vi "PicoScope2000aSetupStreaming.vi"(0 "error in":errorcluster, 1 "Device Info":T1, 2 "handle in":i16, 3 "Acquisition Settings":T3={"Auto Stop"=FALSE, "Desired Sample Interval"=4, "Pre-trigger Samples"=0, "Post-trigger Samples"=1000, "Down-Sample Ratio"=1, "Down-Sample Mode"=0, "Time Units"=2} {"Time Units" items=["Nanoseconds (ns)"=2, "Microseconds (us)"=3, "Milliseconds (ms)"=4, "Seconds (s)"=5]; "Down-Sample Mode" items=["None"=0, "Aggregate"=1, "Decimate"=2, "Average"=4]}, 4 "Buffer and Transfer Settings":T2={"startIndex"=0, "Samples"=1000000, "Down Sample Ratio"=1, "Down-Sample Mode"=0} {"Down-Sample Mode" items=["None"=0, "Aggregate"=1, "Decimate"=2, "Average"=4]; "Down Sample Ratio" step=1; "Samples" format="%_6p"}, 5 "enabled array":i16[](array[numeric]), 10 "Pointers In":u64[][](array[numeric])) -> (11 "Pointer array":u64[][](array[numeric]), 14 "error out":errorcluster, 16 "handle out":i16, 17 "Sample Interval":u32, 19 "sampleIntervalTimeUnits":u32)   [LabVIEW 2010]
doc: "Set up the data buffers and calls RunStreaming to start the device streaming.\nData will be copied from the driver buffers into the corresponding application buffers using the wrapper dll."
uses:
  ps2000aWrap.dll
  ps2000a.dll
panel:
  # "Overview Buffer Size is the size of the temporary buffers used to\nstore data before returning it to the application."
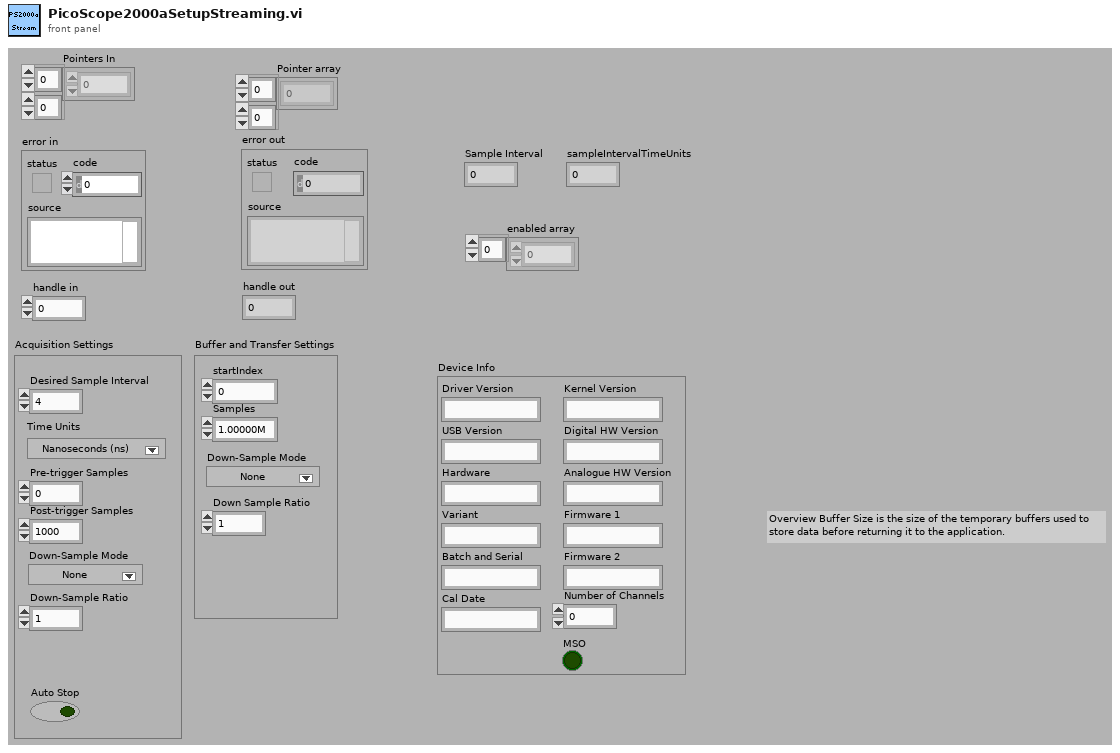
[diagram p1: front panel]
types:
  T1 = cluster{"Driver Version":string, "USB Version":string, "Hardware":string, "Variant":string, "Batch and Serial":string, "Cal Date":string, "Kernel Version":string, "Digital HW Version":string, "Analogue HW Version":string, "Firmware 1":string, "Firmware 2":string, "MSO":bool, "Number of Channels":i16}
  T2 = cluster{"startIndex":u64, "Samples":u64, "Down Sample Ratio":u64, "Down-Sample Mode":u32}
  T3 = cluster{"Auto Stop":bool, "Desired Sample Interval":u32, "Pre-trigger Samples":u32, "Post-trigger Samples":u32, "Down-Sample Ratio":u32, "Down-Sample Mode":i32, "Time Units":u32}
  T4 = cluster{"status":bool, "code":u32, "source":string}
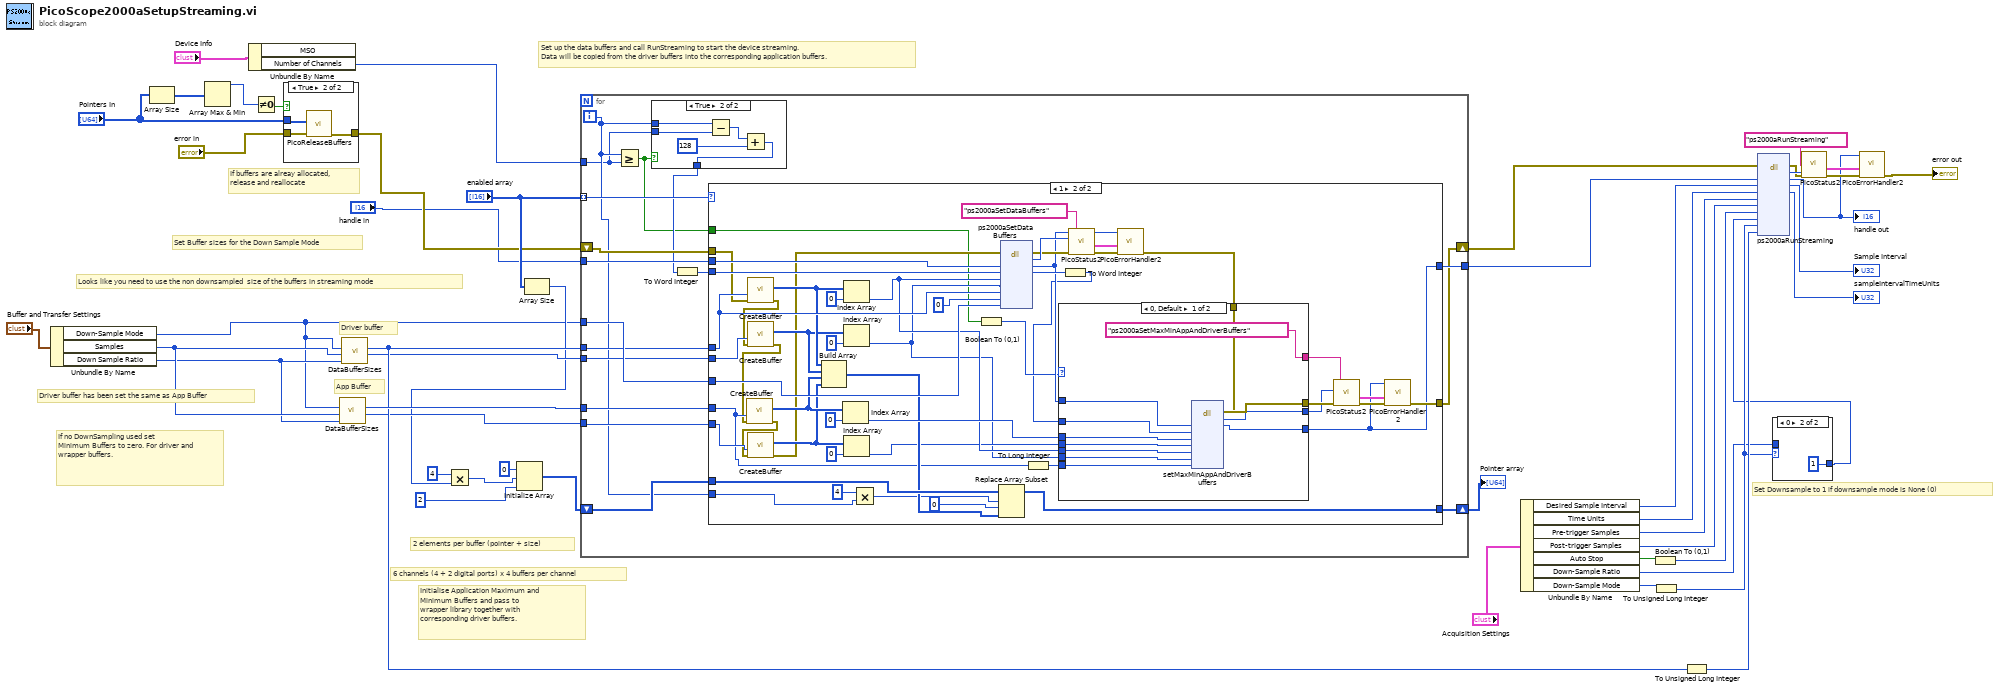
[diagram p0: block diagram]
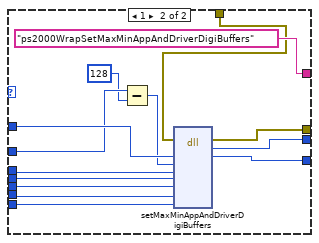
[diagram p6: hidden frame]
diagram:
  # "Set Downsample to 1 if downsample mode is None (0)"
  # "Looks like you need to use the non downsampled  size of the buffers in streaming mode"
  # "If buffers are alreay allocated,\nrelease and reallocate"
  # "2 elements per buffer (pointer + size)"
  # "6 channels (4 + 2 digital ports) x 4 buffers per channel"
  # "App Buffer"
  # "Driver buffer"
  # "Driver buffer has been set the same as App Buffer"
  # "Set Buffer sizes for the Down Sample Mode"
  # "If no DownSampling used set \nMinimum Buffers to zero. For driver and wrapper buffers."
  # "Initialise Application Maximum and\nMinimum Buffers and pass to \nwrapper library together with corresponding driver buffers."
  # "Set up the data buffers and call RunStreaming to start the device streaming.\nData will be copied from the driver buffers into the corresponding application buffers."
  n1 = Unbundle By Name("Buffer and Transfer Settings") -> ("Down-Sample Mode"=w12:u32, "Samples"=w35:u64, "Down Sample Ratio"=w34:u64)
  n2 = Array Size(array="Pointers In") -> (size(s)=w15:i32[])
  n3 = Array Max & Min(array=w15) -> (max value=w14:i32)  [unwired: 3 out]
  n4 = Unbundle By Name("Device Info") -> ("Number of Channels"=w5:i16)  [unwired: 1 out]
  n5 = Not Equal To 0?(x=w14) -> (x != 0?=w19:bool)
  n6 = case shown="True" w19 {
    tunnel: "Pointers In" -> [_ w50]
    tunnel: "error in" -> [w49 w51]
    tunnel: [w49 w52] -> w7
    frame False {
    }
    frame True {
      n7 = call "PicoReleaseBuffers.vi"("error in (no error)"=w51, "Pointer array"=w50) -> ("error out"=w52:errorcluster)  [unwired: 8 in, 1 out]
    }
  }
  n8 = call "DataBufferSizes.vi"("Down Sample Ratio"=w34, "Number of Samples"=w35, "Down-Sample Mode"=w12) -> ("min Buffer Size"=w30:i32, "Max Buffer Size"=w33:i32)  [unwired: 7 in]
  n9 = call "DataBufferSizes.vi"("Down Sample Ratio"=w34, "Number of Samples"=w35, "Down-Sample Mode"=w12) -> ("min Buffer Size"=w31:i32, "Max Buffer Size"=w32:i32)  [unwired: 7 in]
  n10 = Array Size(array="enabled array") -> (size(s)=w23:i32)
  n11 = Multiply(x=4, y=w23) -> (x*y=w24:i32)
  n12 = Initialize Array(u64 0 ("element"), w24, 2 ("dimension size")) -> (w16:u64[][])
  n13 = for {
    tunnel: "enabled array" -> [w61] mode=indexing
    tunnel: "handle in" -> [w69]
    tunnel: w12 -> [w68]
    tunnel: w33 -> [w67]
    tunnel: w32 -> [w66]
    tunnel: w31 -> [w65]
    tunnel: w30 -> [w64]
    tunnel: [w62] -> w26
    shift-right: [w60] -> w20
    shift-left: w7 -> [w59]
    shift-right: [w63] -> w29
    shift-left: w16 -> [w58]
    tunnel: w5 -> [w54]
    i -> [w55]
    n14 = Greater Or Equal?(x=w55, y=w54) -> (x >= y?=w53:bool)
    n15 = case shown="True" w53 {
      tunnel: [w70 w74] -> w56
      tunnel: w55 -> [w70 w72]
      tunnel: w54 -> [_ w71]
      frame False {
      }
      frame True {
        n16 = Subtract(x=w72, y=w71) -> (x-y=w73:i32)
        n17 = Add(x=w73, y=128) -> (x+y=w74:i32)
      }
    }
    n18 = To Word Integer(number=w56) -> (16bit integer=w57:i16)
    n19 = case shown="1" w61 {
      tunnel: w69 -> [w77 w129]
      tunnel: w59 -> [w76 w92]
      tunnel: w57 -> [_ w123]
      tunnel: w67 -> [_ w95]
      tunnel: w66 -> [_ w113]
      tunnel: w65 -> [_ w116]
      tunnel: w64 -> [_ w115]
      tunnel: w68 -> [_ w114]
      tunnel: w58 -> [w78 w107]
      tunnel: [w78 w106] -> w63
      tunnel: w55 -> [_ w103]
      tunnel: [w77 w79] -> w62
      tunnel: [w76 w81] -> w60
      tunnel: w53 -> [_ w86]
      frame 0, Default {
      }
      frame 1 {
        n20 = call "CreateBuffer.vi"("error in (no error)"=w92, "Buffer size"=w113) -> ("error out"=w91:errorcluster, "Pointer and BufferSize"=w111:u64[])  [unwired: 8 in]
        n21 = call "CreateBuffer.vi"("error in (no error)"=w91, "Buffer size"=w116) -> ("error out"=w90:errorcluster, "Pointer and BufferSize"=w110:u64[])  [unwired: 8 in]
        n22 = call "CreateBuffer.vi"("error in (no error)"=w90, "Buffer size"=w95) -> ("error out"=w89:errorcluster, "Pointer and BufferSize"=w109:u64[])  [unwired: 8 in]
        n23 = call "CreateBuffer.vi"("error in (no error)"=w89, "Buffer size"=w115) -> ("error out"=w88:errorcluster, "Pointer and BufferSize"=w108:u64[])  [unwired: 8 in]
        n24 = Build Array(w111, w110, w109, w108) -> (w102:u64[][])
        n25 = Index Array(array=w109, index=0) -> (element=w112:u64)
        n26 = Index Array(array=w111, index=0) -> (element=w105:u64)
        n27 = Index Array(array=w110, index=0) -> (element=w93:u64)
        n28 = Index Array(array=w108, index=0) -> (element=w94:u64)
        n29 = Multiply(x=4, y=w103) -> (x*y=w101:i32)
        n30 = Boolean To (0,1)(Boolean=w86) -> (0, 1=w85:i16)
        n31 = Replace Array Subset(array=w107, new element=w102, index (row)=w101, index (col)=0 ("disabled index (row)")) -> (w106:u64[][])
        n32 = dll-call lib="ps2000a.dll" fn="ps2000aSetDataBuffers" ("ps3000.dll:_ps3000_open_unit@0")(error in=w88, "handle"=w129, "channel"=w123, "bufferMax"=w105, "bufferMin"=w93, "bufferLth"=w113, "segmentIndex"=u32 0, "downSampleRatioMode"=w114) -> (error out=w127:errorcluster, "PICO_STATUS"=w128:u32, "handle"=w97:i16, "channel"=w124:i16)  [unwired: 7 in, 1 out]
        n33 = To Long Integer(number=w95) -> (32bit integer=w96:i32)
        n34 = To Word Integer(number=w124) -> (16bit integer=w84:i16)
        n35 = call "PicoStatus2.vi"("PICO source"="ps2000aSetDataBuffers" ("source"), "Error in"=w127, "PICO STATUS"=w128) -> ("error out"=w99:errorcluster, "PICO_STATUS out"=w83:T4)  [unwired: 5 in]
        n36 = call "PicoErrorHandler2.vi"("error in (no error)"=w99, "PICO_STATUS in"=w83, "handle In"=w97) -> ("error out"=w98:errorcluster)  [unwired: 8 in]
        n37 = case shown="0, Default" w85 {
          tunnel: w84 -> [w130 w143]
          tunnel: [w141 w154] -> w122
          tunnel: [w140 w153] -> w121
          tunnel: w112 -> [w139 w147]
          tunnel: w105 -> [w138 w145]
          tunnel: [w137 w150] -> w79
          tunnel: w98 -> [w136 w152]
          tunnel: w97 -> [w135 w149]
          tunnel: w96 -> [w134 w151]
          tunnel: w94 -> [w133 w146]
          tunnel: w93 -> [w132 w148]
          tunnel: ["ps2000aSetMaxMinAppAndDriverBuffers" ("source") "ps2000WrapSetMaxMinAppAndDriverDigiBuffers" ("source")] -> w87
          frame 0, Default {
            n38 = dll-call lib="ps2000aWrap.dll" fn="setMaxMinAppAndDriverBuffers"(error in=w136, "handle"=w135, "channel"=w130, "appMaxBuffer"=w139, "appMinBuffer"=w133, "driverMaxBuffer"=w138, "driverMinBuffer"=w132, "bufferLength"=w134) -> (error out=w141:errorcluster, "status"=w140:u32, "handle"=w137:i16)  [unwired: 8 in, 1 out]
          }
          frame 1 {
            n39 = Subtract(x=w143, y=i16 128) -> (x-y=w144:i16)
            n40 = dll-call lib="ps2000aWrap.dll" fn="setMaxMinAppAndDriverDigiBuffers" ("setMaxMinAppAndDriverBuffers")(error in=w152, "handle"=w149, "digiPort"=w144, "appMaxDigiBuffer"=w147, "appMinDigiBuffer"=w146, "driverMaxDigiBuffer"=w145, "driverMinDigiBuffer"=w148, "bufferLength"=w151) -> (error out=w154:errorcluster, "status"=w153:u32, "handle"=w150:i16)  [unwired: 8 in, 1 out]
          }
        }
        n41 = call "PicoStatus2.vi"("PICO source"=w87, "Error in"=w122, "PICO STATUS"=w121) -> ("error out"=w82:errorcluster, "PICO_STATUS out"=w80:T4)  [unwired: 5 in]
        n42 = call "PicoErrorHandler2.vi"("error in (no error)"=w82, "PICO_STATUS in"=w80, "handle In"=w79) -> ("error out"=w81:errorcluster)  [unwired: 8 in]
      }
    }
  }
  "Pointer array" <- w29
  n43 = Unbundle By Name("Acquisition Settings") -> ("Desired Sample Interval"=w43:u32, "Time Units"=w37:u32, "Pre-trigger Samples"=w42:u32, "Post-trigger Samples"=w41:u32, "Auto Stop"=w40:bool, "Down-Sample Ratio"=w10:u32, "Down-Sample Mode"=w38:i32)
  n44 = Boolean To (0,1)(Boolean=w40) -> (0, 1=w44:i16)
  n45 = To Unsigned Long Integer(number=w38) -> (unsigned 32bit integer=w11:u32)
  n46 = To Unsigned Long Integer(number=w32) -> (unsigned 32bit integer=w13:u32)
  n47 = case shown="0" w11 {
    tunnel: [w156 u32 1 ("Down-Sample Ratio")] -> w9
    tunnel: w10 -> [w156 _]
    frame Default {
    }
    frame 0 {
    }
  }
  n48 = dll-call lib="ps2000a.dll" fn="ps2000aRunStreaming" ("ps5000a.dll:_ps3000_open_unit@0")(error in=w20, "handle"=w26, "sampleInterval"=w43, "sampleIntervalTimeUnits"=w37, "maxPreTriggerSamples"=w42, "maxPostTriggerSamples"=w41, "autoStop"=w44, "downSampleRatio"=w9, "downSampleRatioMode"=w11, "overviewBufferSize"=w13) -> (error out=w47:errorcluster, "PICO_STATUS"=w48:u32, "handle"=w1:i16, "sampleInterval"=→"Sample Interval":u32, "sampleIntervalTimeUnits"=→"sampleIntervalTimeUnits":u32)  [unwired: 8 in, 1 out]
  "handle out" <- w1
  n49 = call "PicoStatus2.vi"("PICO source"="ps2000aRunStreaming" ("source"), "Error in"=w47, "PICO STATUS"=w48) -> ("error out"=w4:errorcluster, "PICO_STATUS out"=w3:T4)  [unwired: 5 in]
  n50 = call "PicoErrorHandler2.vi"("error in (no error)"=w4, "PICO_STATUS in"=w3, "handle In"=w1) -> ("error out"=→"error out":errorcluster)  [unwired: 8 in]
